vi "iXonEMCCD_Close.vi"() -> ()   [LabVIEW 2025]
panel:
  out "Shut Down ？":bool
  out "DLL error code":u32
  out "error out":errorcluster
  in  "error in (no error)":errorcluster
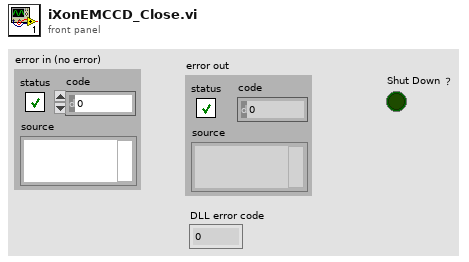
[diagram p1: front panel]
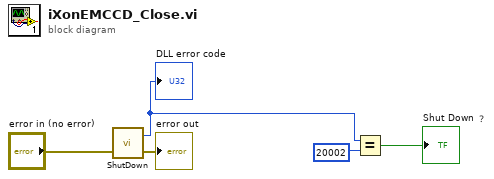
[diagram p0: block diagram]
diagram:
  n1 = call "ShutDown.vi"("error in (no error)"="error in (no error)") -> ("error out"=→"error out":errorcluster, "DLL error code"=w2:u32)  [unwired: 1 in]
  "DLL error code" <- w2
  n2 = Equal?(x=w2, y=u32 20002) -> (x = y?=→"Shut Down ？":bool)
